vi "pH edit buffer list.vi"(3 "index":i32) -> (1 "Buffers out":T1(array[cluster]) {"V/T" format="%.2f"; "Buffer" format="%.2f"})   [LabVIEW 2015]
uses:
  DAQ configuration/Sensor buffer command.ctl
panel:
  in  "Cancel Button":bool
  in  "OK Button":bool
  in  "Buffers":T1(array[cluster]) {"V/T" format="%.2f"; "Buffer" format="%.2f"}
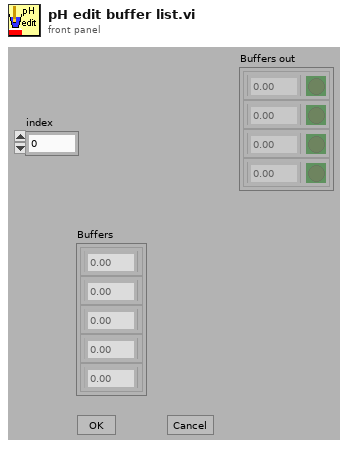
[diagram p1: front panel]
types:
  T1 = cluster{"Buffer":dbl, "Calibrated":bool, "V/T":dbl}[]
  T2 = typedef "Sensor buffer command.ctl" = enum16{"read average", "read recent", "read all", "write", "set buffer size", "Read channel config", "Write channel config", "clear"}
  T3 = typedef "Channel config.ctl" = cluster{"Channel Indices":T4[], "AI Max voltage":dbl[], "Calibration matrix":T5}
  T4 = typedef "channel identifier.ctl" = u16
  T5 = typedef "calib array.ctl" = T6[]
  T6 = typedef "conversion.ctl" = cluster{"conversion matrix":sgl[][], "units":string, "name":string, "scale type":T7, "offset (volts)":dbl, "second channel":i8, "correspondence table":T8, "offset (physical units)":dbl, "pH scale":T9, "D.O.":T10, "Photometer data":T11}
  T7 = typedef "scale type.ctl" = enum16{"Volts", "Polynomial", "Correspondence Table", "pH", "Dissolved Oxygen", "Quadratic", "Photometer"}
  T8 = typedef "correspondence table.ctl" = cluster{"physical units":dbl, "volts":dbl}[]
  T9 = typedef "pH scale.ctl" = cluster{"Buffers":cluster{"Buffer":dbl, "Calibrated":bool, "V/T":dbl}[], "Temperature":dbl}
  T10 = typedef "DO scale.ctl" = cluster{"Temperature":dbl, "K":dbl, "barometric pressure":dbl}
  T11 = typedef "Photometer calibration data.ctl" = cluster{"Dark Voltage":dbl, "Blank Voltage":dbl, "Standards":cluster{"Concentration":dbl, "Voltage":dbl}[]}
  T12 = cluster{"Buffer":dbl, "Calibrated":bool, "V/T":dbl}
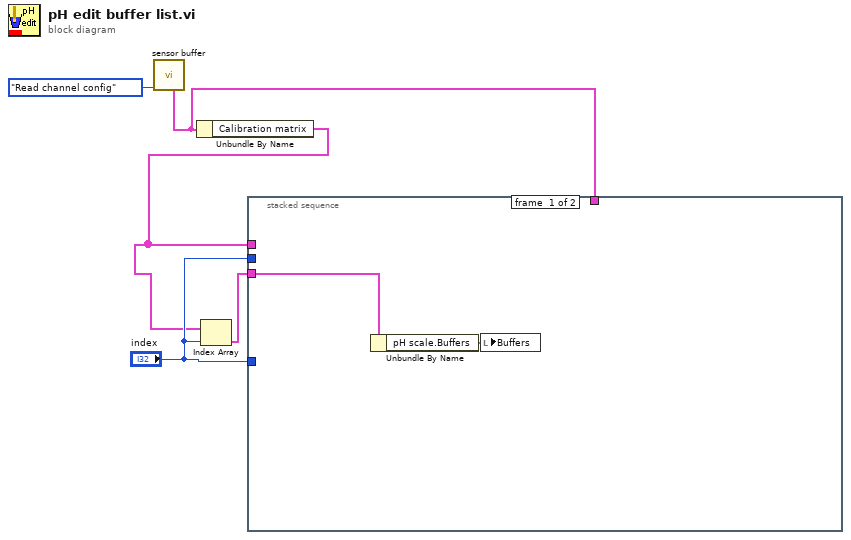
[diagram p0: block diagram]
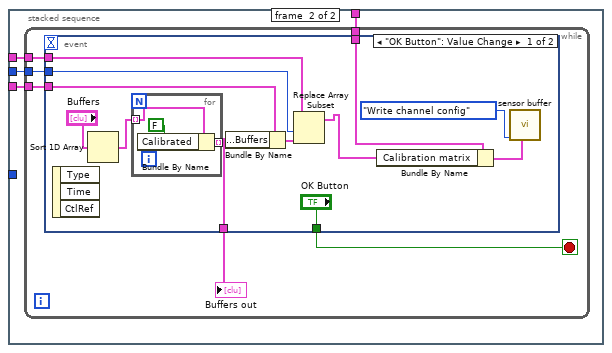
[diagram p2: hidden frame]
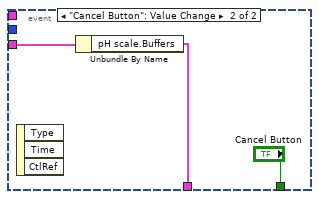
[diagram p3: hidden frame]
diagram:
  n1 = call "sensor buffer.vi"("command"=Sensor_buffer_command."Read channel config") -> ("Channel Config out"=w1:T3)  [unwired: 6 in, 4 out]
  n2 = Unbundle By Name(w1) -> ("Calibration matrix"=w2:T5)
  n3 = Index Array(array=w2, index="index") -> (element=w5:T6)
  n4 = stacked-sequence {
    tunnel: "index" -> [_ _]
    tunnel: w5 -> [w6 w11]
    tunnel: w2 -> [_ w10]
    tunnel: "index" -> [_ w9]
    tunnel: w1 -> [_ w8]
    frame #0 {
      n5 = Unbundle By Name(w6) -> ("pH scale.Buffers"=w7:T1)
      n6 = local write "Buffers"(w7) -> ()
    }
    frame #1 {
      n7 = while {
        tunnel: w11 -> [w17]
        tunnel: w10 -> [w16]
        tunnel: w9 -> [w15]
        tunnel: w8 -> [w12]
        stop <- w14 stop-if-true
        n8 = event shown="[0] \"OK Button\": Value Change" {
          selector: _ -> [_ _]
          dyn-events: _ -> [_ _]
          timeout: _ -> [_ _]
          tunnel: w17 -> [w29 w34]
          tunnel: w16 -> [w28 _]
          tunnel: w15 -> [w27 _]
          tunnel: ["OK Button" "Cancel Button"] -> w14
          tunnel: [w24 w33] -> w13
          tunnel: w12 -> [w18 _]
          event "OK Button": Value Change {
            n9 = event-data() -> ()  [unwired: 1 in, 3 out]
            n10 = Sort 1D Array(array="Buffers") -> (sorted array=w22:T1)
            n11 = for {
              tunnel: w22 -> [w32] mode=indexing
              tunnel: [w30] -> w24 mode=indexing
              n12 = Bundle By Name(cluster=w32, "Calibrated"=FALSE) -> (w30:T12)
            }
            n13 = Bundle By Name(cluster=w29, "pH scale.Buffers"=w24) -> (w25:T6)
            n14 = Replace Array Subset(array=w28, new element=w25, index=w27) -> (w19:T5)
            n15 = Bundle By Name(cluster=w18, "Calibration matrix"=w19) -> (w21:T3)
            n16 = call "sensor buffer.vi"("Channel Config"=w21, "command"=Sensor_buffer_command."Write channel config") -> ()  [unwired: 5 in, 5 out]
          }
          event "Cancel Button": Value Change {
            n17 = event-data() -> ()  [unwired: 1 in, 3 out]
            n18 = Unbundle By Name(w34) -> ("pH scale.Buffers"=w33:T1)
          }
        }
        "Buffers out" <- w13
      }
    }
  }
